vi "PC_SVG to TDVM with trigger.vi"() -> ()   [LabVIEW 2021]
uses:
  Signal Voltage Generation/Typedefs/Signal Generation Settings.ctl
  Signal Voltage Generation/Typedefs/Generation Types.ctl
  Signal Voltage Generation/Typedefs/Single Tone Settings.ctl
  Signal Voltage Generation/Typedefs/Waveform Type.ctl
  Signal Voltage Generation/Typedefs/Tone Settings.ctl
  Time Domain Measurement/Typedefs/Time Domain Measurements.ctl
  Time Domain Measurement/Typedefs/Range and Terminal Settings.ctl
  Time Domain Measurement/Typedefs/Specific Channel Settings.ctl
  Time Domain Measurement/Typedefs/Execution Settings.ctl
  Common/Typedefs/Execution Options - Measure.ctl
  Time Domain Measurement/Typedefs/Timing & Trigger Settings.ctl
  Time Domain Measurement/Typedefs/Timing Settings.ctl
  Time Domain Measurement/Typedefs/Trigger Settings.ctl
  Time Domain Measurement/DAQ_Time Domain Measurement.lvlib
  Signal Voltage Generation/DAQ_Signal Voltage Generation.lvlib
panel:
  in  "Range and Terminal Settings":T1={"Global Settings"={"Min Range(V)"=-10.0, "Max Range(V)"=10.0, "Terminal Configuration"=10083}, "Specific Channel Settings"=[{"Active Channels"="Dev1/ai0", "Min Range"=-5.0, "Max Range"=5.0, "Terminal Configuration"=10106}, {"Active Channels"="Dev1/ai2", "Min Range"=-1.0, "Max Range"=1.0, "Terminal Configuration"=10106}]} {"Specific Channel Settings"."Terminal Configuration" items=["RSE"=10083, "NRSE"=10078, "Differential"=10106]; "Specific Channel Settings"."Max Range" format="%.2p"; "Specific Channel Settings"."Min Range" format="%.2p"; "Global Settings"."Terminal Configuration" items=["RSE"=10083, "NRSE"=10078, "Differential"=10106]; "Global Settings"."Max Range(V)" format="%.2p"; "Global Settings"."Min Range(V)" format="%.2p"}
  out "Time Domain Measurements":T3={"Mean DC Voltage (V)"=[0.9995928813147406, 1.000286334378455, 0.5009882754593022, 0.49885920760939795, 0.49711856447168623], "Vpp Amplitude(V)"=[2.000122637627838, 2.0007247673921813, 1.0011645102829598, 0.9997176535335253, 0.995850273739072], "Voltage Frequency(Hz)"=[100.00206474752596, 99.99949264783776, 100.01759743361525, 100.00447770140465, 99.99608341298507], "Voltage Waveform Period (s)"=[0.009999793529510498, 0.010000050735473632, 0.00999824056625366, 0.009999552249908446, 0.010000391674041747], "Voltage Waveform duty cycle (%)"=[50.00099470284969, 50.00332544546951, 49.9961140471273, 49.99776162615618, 49.99962045248796]} {"Voltage Waveform duty cycle (%)" format="%.2p"; "Voltage Waveform Period (s)" format="%.2p"; "Voltage Frequency(Hz)" format="%.2p"; "Vpp Amplitude(V)" format="%.2p"; "Mean DC Voltage (V)" format="%.2p"}
  out "Measured Voltage Waveforms":waveform(dbl)[](graph)=[{"t0"=timestamp(3825153874.8210855 s since 1904-01-01), "dt"=9.999999999999999e-05, "Y"=array[1000 elements], "attributes"=variant("NI_ChannelName"=variant(string "Dev1/ai0"), "NI_UnitDescription"=variant(string "Volts"))}, {"t0"=timestamp(3825153874.8210964 s since 1904-01-01), "dt"=9.999999999999999e-05, "Y"=array[1000 elements], "attributes"=variant("NI_ChannelName"=variant(string "Dev1/ai1"), "NI_UnitDescription"=variant(string "Volts"))}, {"t0"=timestamp(3825153874.8211074 s since 1904-01-01), "dt"=9.999999999999999e-05, "Y"=array[1000 elements], "attributes"=variant("NI_ChannelName"=variant(string "Dev1/ai2"), "NI_UnitDescription"=variant(string "Volts"))}, {"t0"=timestamp(3825153874.8211184 s since 1904-01-01), "dt"=9.999999999999999e-05, "Y"=array[1000 elements], "attributes"=variant("NI_ChannelName"=variant(string "Dev1/ai3"), "NI_UnitDescription"=variant(string "Volts"))}, {"t0"=timestamp(3825153874.8211293 s since 1904-01-01), "dt"=9.999999999999999e-05, "Y"=array[1000 elements], "attributes"=variant("NI_ChannelName"=variant(string "Dev1/ai4"), "NI_UnitDescription"=variant(string "Volts"))}] caption="Voltage Waveforms"
  out "Generated Voltage Waveforms":waveform(dbl)[](graph)=[{"t0"=timestamp(0 s since 1904-01-01), "dt"=1e-05, "Y"=array[10000 elements]}, {"t0"=timestamp(0 s since 1904-01-01), "dt"=1e-05, "Y"=array[10000 elements]}, {"t0"=timestamp(0 s since 1904-01-01), "dt"=1e-05, "Y"=array[10000 elements]}, {"t0"=timestamp(0 s since 1904-01-01), "dt"=1e-05, "Y"=array[10000 elements]}]
  in  "Signal Generation Settings":T4={"Generation Type"=enum."Single Tone", "Generation Time (s)"=0.1, "Voltage Offset (v)"=1.0, "Single Tone Settings"={"Waveform Type"=enum."Sine Wave", "Frequency (Hz)"=100.0, "Amplitude (V)"=1.0, "Duty Cycle (%)"=20.0}, "Multi Tone Settings"=[]} {"Voltage Offset (v)" format="%.2p"; "Generation Time (s)" format="%.2p"; "Multi Tone Settings"."Amplitude (V)" format="%#.2p"; "Multi Tone Settings"."Frequency (Hz)" format="%#.2p"; "Single Tone Settings"."Duty Cycle (%)" format="%#.2p"; "Single Tone Settings"."Amplitude (V)" format="%#.2p"; "Single Tone Settings"."Frequency (Hz)" format="%#.2p"}
  out "error out":errorcluster
  # "Min. Range(V)"
  # "Max. Range(V)"
  # "Terminal Configuration"
  # "Physical Channel Name"
  # "Frequency (Hz)"
  # "Amplitude (V)"
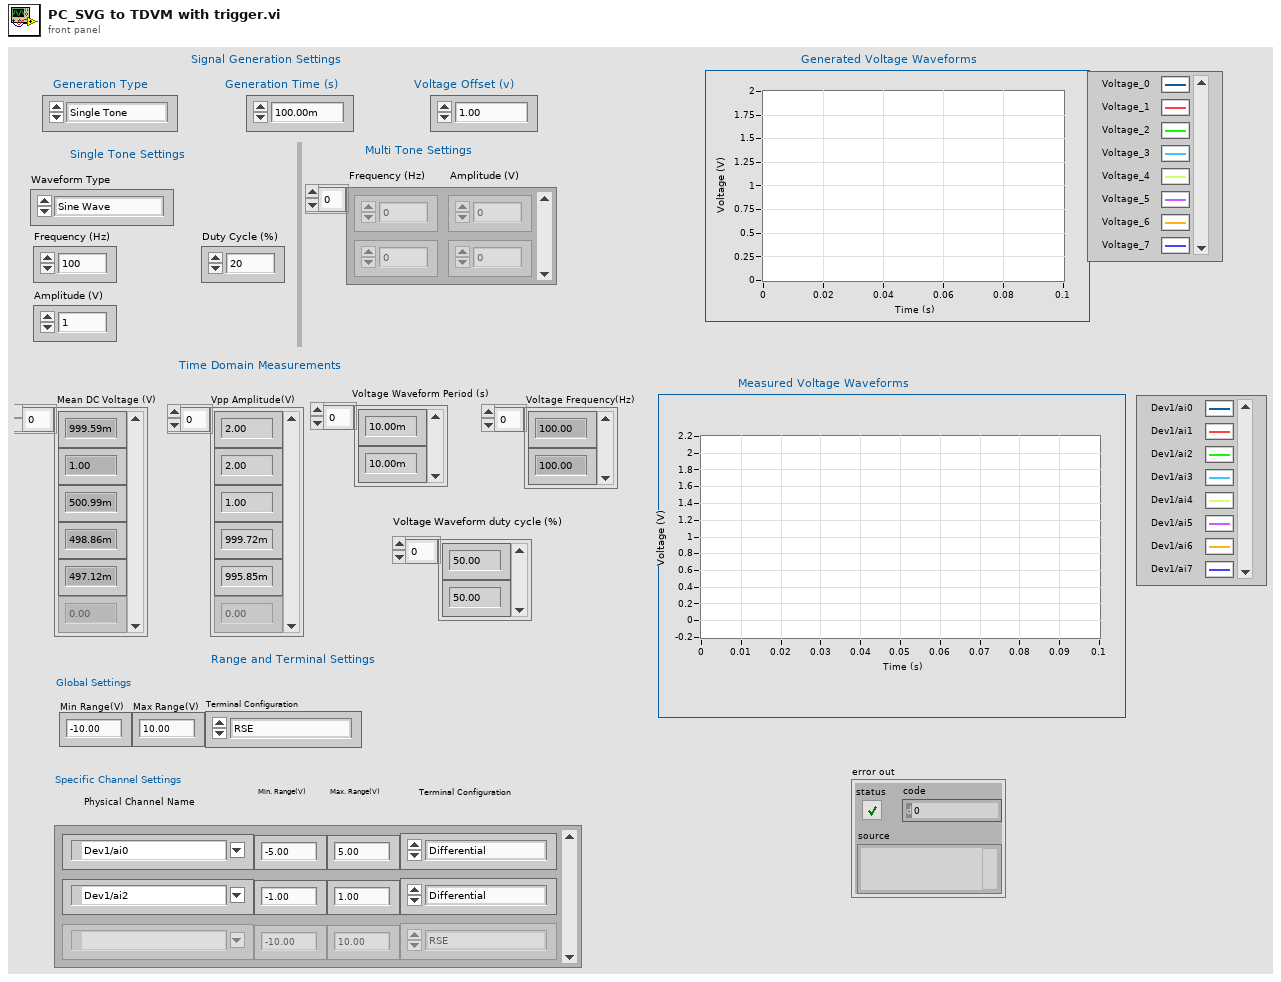
[diagram p1: front panel]
types:
  T1 = typedef "DAQ_Time Domain Measurement.lvlib/Range and Terminal Settings.ctl" = cluster{"Global Settings":cluster{"Min Range(V)":dbl, "Max Range(V)":dbl, "Terminal Configuration":i32}, "Specific Channel Settings":T2[]}
  T2 = typedef "DAQ_Time Domain Measurement.lvlib/Specific Channel Settings.ctl" = cluster{"Active Channels":tag, "Min Range":dbl, "Max Range":dbl, "Terminal Configuration":i32}
  T3 = typedef "DAQ_Time Domain Measurement.lvlib/Time Domain Measurements.ctl" = cluster{"Mean DC Voltage (V)":dbl[], "Vpp Amplitude(V)":dbl[], "Voltage Frequency(Hz)":dbl[], "Voltage Waveform Period (s)":dbl[], "Voltage Waveform duty cycle (%)":dbl[]}
  T4 = typedef "DAQ_Signal Voltage Generation.lvlib/Signal Generation Settings.ctl" = cluster{"Generation Type":T5, "Generation Time (s)":dbl, "Voltage Offset (v)":dbl, "Single Tone Settings":T6, "Multi Tone Settings":T8[]}
  T5 = typedef "DAQ_Signal Voltage Generation.lvlib/Generation Types.ctl" = enum16{"Single Tone", "Multi Tone"}
  T6 = typedef "DAQ_Signal Voltage Generation.lvlib/Single Tone Settings.ctl" = cluster{"Waveform Type":T7, "Frequency (Hz)":dbl, "Amplitude (V)":dbl, "Duty Cycle (%)":dbl}
  T7 = typedef "DAQ_Signal Voltage Generation.lvlib/Waveform Type.ctl" = enum16{"Sine Wave", "Square Wave"}
  T8 = typedef "DAQ_Signal Voltage Generation.lvlib/Tone Settings.ctl" = cluster{"Frequency (Hz)":dbl, "Amplitude (V)":dbl}
  T9 = typedef "DAQ_Time Domain Measurement.lvlib/Timing & Trigger Settings.ctl" = cluster{"Timing Settings":T10, "Trigger Settings":T11}
  T10 = typedef "DAQ_Time Domain Measurement.lvlib/Timing Settings.ctl" = cluster{"Sample Clock Source":tag, "Sample Rate(Hz)":dbl, "Number of Samples":i32, "Sample Timing Engine":enum16{"te0", "te1", "ai", "Auto"}}
  T11 = typedef "DAQ_Time Domain Measurement.lvlib/Trigger Settings.ctl" = cluster{"Trigger Type":enum16{"No Trigger", "Digital Start"}, "Digital Start Trigger Source":tag, "Digital Start Trigger Edge":i32}
  T12 = typedef "DAQ_Time Domain Measurement.lvlib/Execution Settings.ctl" = cluster{"Execution option":T13, "Skip Analysis?":bool}
  T13 = typedef "Execution Options - Measure.ctl" = enum16{"Configure & Measure", "Configure only", "Measure only"}
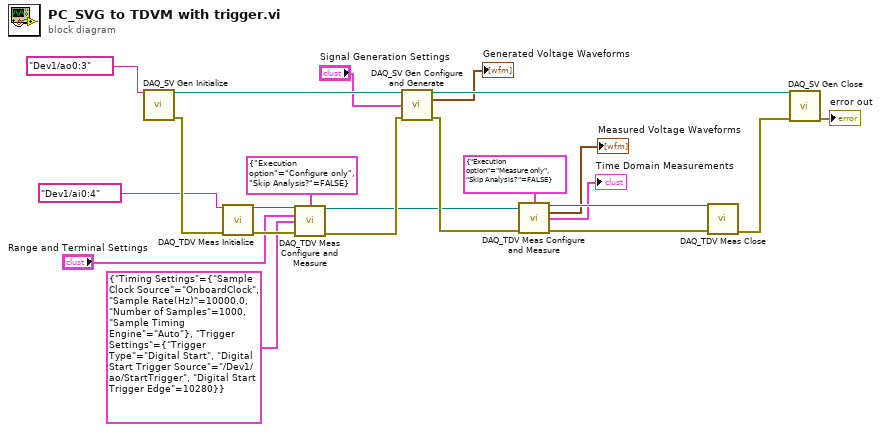
[diagram p0: block diagram]
diagram:
  n1 = call "DAQ_SV Gen Initialize.vi"("Physical Channels"=tag "Dev1/ao0:3") -> ("DAQmx Task Out"=w22:refnum<k21>, "error out"=w20:errorcluster)  [unwired: 13 in]
  n2 = call "DAQ_TDV Meas Initialize.vi"("Physical Channels"=tag "Dev1/ai0:4", "error in"=w20) -> ("DAQmx Task Out"=w11:refnum<k21>, "error out"=w19:errorcluster)  [unwired: 12 in]
  n3 = call "DAQ_TDV Meas Configure and Measure.vi"("DAQmx Task In"=w11, "Execution Settings"=T12 {"Execution option"=enum."Configure only", "Skip Analysis?"=FALSE}, "Range and Terminal Settings"="Range and Terminal Settings", "Timing and Trigger Settings"=T9 {"Timing Settings"={"Sample Clock Source"="OnboardClock", "Sample Rate(Hz)"=10000.0, "Number of Samples"=1000, "Sample Timing Engine"=enum."Auto"}, "Trigger Settings"={"Trigger Type"=enum."Digital Start", "Digital Start Trigger Source"="/Dev1/ao/StartTrigger", "Digital Start Trigger Edge"=10280}}, "error in"=w19) -> ("DAQmx Task Out"=w10:refnum<k21>, "error out"=w17:errorcluster)  [unwired: 6 in, 3 out]
  n4 = call "DAQ_SV Gen Configure and Generate.vi"("DAQmx Task In"=w22, "Signal Generation Settings"="Signal Generation Settings", "error in"=w17) -> ("DAQmx Task Out"=w21:refnum<k21>, "Generated Voltage Waveforms"=→"Generated Voltage Waveforms":waveform(dbl)[], "error out"=w16:errorcluster)  [unwired: 10 in]
  n5 = call "DAQ_TDV Meas Configure and Measure.vi"("DAQmx Task In"=w10, "Execution Settings"=T12 {"Execution option"=enum."Measure only", "Skip Analysis?"=FALSE}, "error in"=w16) -> ("DAQmx Task Out"=w9:refnum<k21>, "Voltage Waveforms"=→"Measured Voltage Waveforms":waveform(dbl)[], "Time Domain Measurements"=→"Time Domain Measurements":T3, "error out"=w15:errorcluster)  [unwired: 8 in, 1 out]
  n6 = call "DAQ_TDV Meas Close.vi"("DAQmx Task In"=w9, "error in"=w15) -> ("error out"=w14:errorcluster)  [unwired: 13 in]
  n7 = call "DAQ_SV Gen Close.vi"("DAQmx Task In"=w21, "error in"=w14) -> ("error out"=→"error out":errorcluster)  [unwired: 13 in]
